vi "NF90 command interface.vi"(0 "port number in":refnum<visa-resource-name>, 1 "scaling (steps/cm)":sgl=2000.0 min=-1048575 max=1048575 step=1 format="%.2f", 2 "time out (ms)":u32=30000, 5 "commands":T2, 7 "axis":T1, 9 "enable?":bool, 11 "Error In":errorcluster, 12 "Distance":sgl format="%.2f", 13 "Speed":sgl=1.0 format="%.2f", 14 "Acceleration":u8=1 min=1 max=50 step=1) -> (4 "port number out":refnum<visa-resource-name>, 6 "Response":string, 8 "Position":sgl format="%.2f", 10 "timed out":bool, 15 "Error Out":errorcluster)   [LabVIEW 2015]
uses:
  NF90 commands.ctl
  Axis.ctl
panel:
  out "Command String":string
  in  "code":string[](array[string])=["I", "S", "A", "B", "Q", "R", "N", "V", "C", "F", "G", "H"]
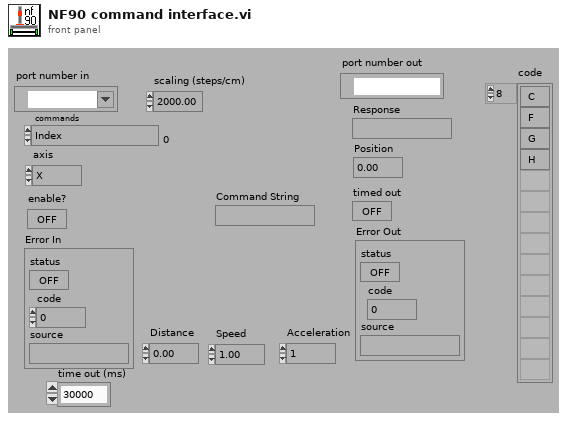
[diagram p1: front panel]
types:
  T1 = typedef "Axis.ctl" = enum16{"X", "Y", "Z"}
  T2 = typedef "NF90 commands.ctl" = enum16{"Index", "Speed", "Acceleration", "Backlash", "Quit", "Run", "Null indexes", "Verify status", "Clear program", "Computer Control", "Go", "Put Controller on Hold", "Position"}
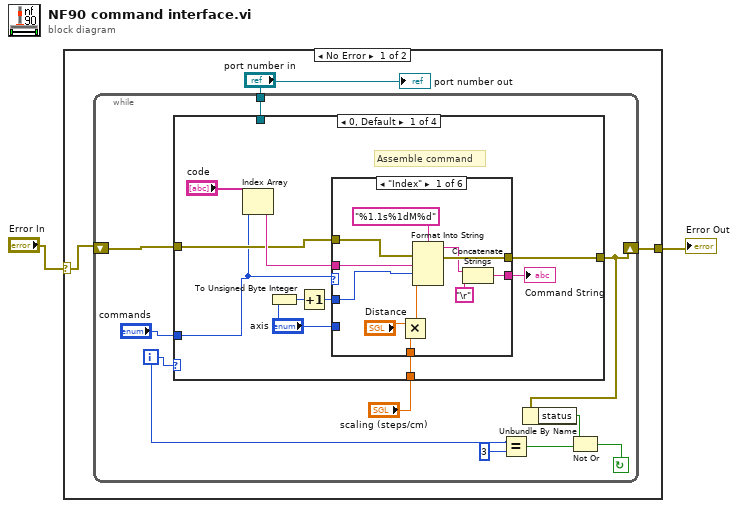
[diagram p0: block diagram]
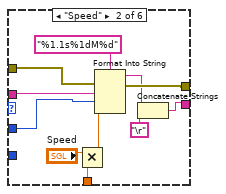
[diagram p2: hidden frame]
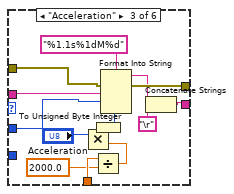
[diagram p3: hidden frame]
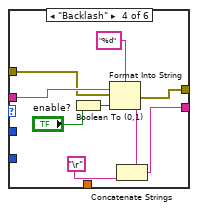
[diagram p4: hidden frame]
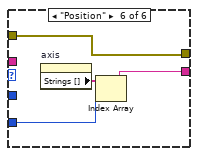
[diagram p6: hidden frame]
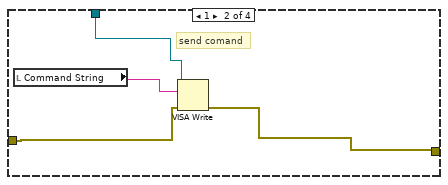
[diagram p7: hidden frame]
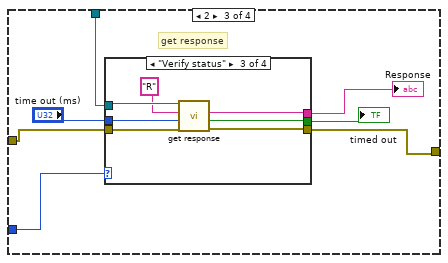
[diagram p8: hidden frame]
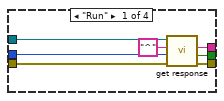
[diagram p9: hidden frame]
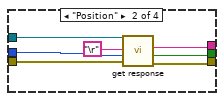
[diagram p10: hidden frame]
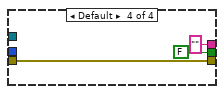
[diagram p11: hidden frame]
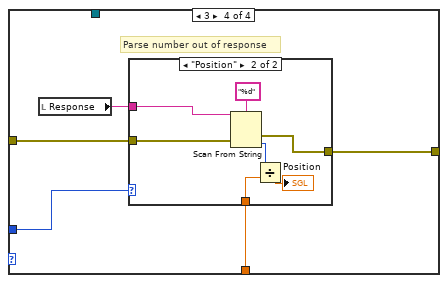
[diagram p12: hidden frame]
diagram:
  n1 = case shown="No Error" "Error In" {
    selector: "Error In" -> [w3 w125]
    tunnel: [w4 w125] -> w2
    frame No Error {
      n2 = while {
        tunnel: "port number in" -> [w13]
        shift-left: w3 -> [w14]
        shift-right: [w12] -> w4
        i -> [w15]
        stop <- w7 continue-if-true
        n3 = case shown="0, Default" w15 {
          tunnel: w14 -> [w20 w78 w86 w116]
          tunnel: [w19 w77 w84 w115] -> w12
          tunnel: w13 -> [_ w80 w87 _]
          tunnel: "commands" -> [w17 _ w83 w114]
          tunnel: "scaling (steps/cm)" -> [w16 _ _ w112]
          frame 0, Default {
            # "Assemble command"
            n4 = Index Array(array="code", index=w17) -> (element=w24:string)
            n5 = To Unsigned Byte Integer(number="axis") -> (unsigned 8bit integer=w18:u8)
            n6 = Increment(x=w18) -> (x+1=w21:u8)
            n7 = case shown="\"Index\"" w17 {
              tunnel: w24 -> [w35 w44 w58 w64 w72 _]
              tunnel: [w29 w39 w54 w69 w72 w73] -> w23
              tunnel: w21 -> [w34 w43 w57 _ _ _]
              tunnel: w20 -> [w33 w45 w59 w63 w71 w76]
              tunnel: [w32 w42 w60 w62 w71 w76] -> w19
              tunnel: "axis" -> [_ _ _ _ _ w74]
              tunnel: w16 -> [w26 w37 w51 _ _ _]
              frame "Index" {
                n8 = Multiply(x="Distance", y=w26) -> (x*y=w28:sgl)
                n9 = Format Into String(format string="%1.1s%1dM%d" ("Format String"), error in=w33, w35, w34, w28) -> (resulting string=w30:string, error out=w32:errorcluster)  [unwired: 1 in]
                n10 = Concatenate Strings(w30, "\r") -> (w29:string)
              }
              frame "Speed" {
                n11 = Multiply(x="Speed", y=w37) -> (x*y=w38:sgl)
                n12 = Format Into String(format string="%1.1s%1dM%d" ("Format String"), error in=w45, w44, w43, w38) -> (resulting string=w40:string, error out=w42:errorcluster)  [unwired: 1 in]
                n13 = Concatenate Strings(w40, "\r") -> (w39:string)
              }
              frame "Acceleration" {
                n14 = Divide(x=w51, y=sgl 2000.0) -> (x/y=w49:sgl)
                n15 = Multiply(x="Acceleration", y=w49) -> (x*y=w53:sgl)
                n16 = To Unsigned Byte Integer(number=w53) -> (unsigned 8bit integer=w48:u8)
                n17 = Format Into String(format string="%1.1s%1dM%d" ("Format String"), error in=w59, w58, w57, w48) -> (resulting string=w55:string, error out=w60:errorcluster)  [unwired: 1 in]
                n18 = Concatenate Strings(w55, "\r") -> (w54:string)
              }
              frame "Backlash" {
                n19 = Boolean To (0,1)(Boolean="enable?") -> (0, 1=w68:i16)
                n20 = Format Into String(format string="%d" ("Format String"), initial string=w64, error in=w63, w68) -> (resulting string=w65:string, error out=w62:errorcluster)
                n21 = Concatenate Strings(w65, "\r") -> (w69:string)
              }
              frame "Quit".."Put Controller on Hold", Default {
              }
              frame "Position" {
                n22 = property on="axis" class="Enum (strict)"() -> ("Strings []"=w75:string[])  [unwired: 2 in, 2 out]
                n23 = Index Array(array=w75, index=w74) -> (element=w73:string)
              }
            }
            "Command String" <- w23
          }
          frame 1 {
            # "send comand"
            n24 = local read "Command String"() -> (w79:string)
            n25 = VISA Write(VISA resource name=w80, write buffer=w79, error in (no error)=w78) -> (error out=w77:errorcluster)  [unwired: 2 out]
          }
          frame 2 {
            # "get response"
            n26 = case shown="\"Verify status\"" w83 {
              tunnel: w87 -> [w94 w101 w108 _]
              tunnel: w86 -> [w93 w100 w104 w111]
              tunnel: [w92 w98 w107 "" ("response")] -> w85
              tunnel: [w91 w99 w106 w111] -> w84
              tunnel: "time out (ms)" -> [w89 w96 w105 _]
              tunnel: [w88 w95 w103 FALSE ("timed out")] -> w81
              frame "Run" {
                n27 = call "get response.vi"("error in (no error)"=w93, "time out (ms)"=w89, "end char"="^", "port number"=w94) -> ("error out"=w91:errorcluster, "timed out"=w88:bool, "response"=w92:string)  [unwired: 4 in, 1 out]
              }
              frame "Position" {
                n28 = call "get response.vi"("error in (no error)"=w100, "time out (ms)"=w96, "end char"="\r", "port number"=w101) -> ("error out"=w99:errorcluster, "timed out"=w95:bool, "response"=w98:string)  [unwired: 4 in, 1 out]
              }
              frame "Verify status" {
                n29 = call "get response.vi"("error in (no error)"=w104, "time out (ms)"=w105, "end char"="R", "port number"=w108) -> ("error out"=w106:errorcluster, "timed out"=w103:bool, "response"=w107:string)  [unwired: 4 in, 1 out]
              }
              frame Default {
              }
            }
            "timed out" <- w81
            "Response" <- w85
          }
          frame 3 {
            # "Parse number out of response"
            n30 = local read "Response"() -> (w113:string)
            n31 = case shown="\"Position\"" w114 {
              tunnel: w116 -> [w117 w123]
              tunnel: [w117 w122] -> w115
              tunnel: w113 -> [_ w121]
              tunnel: w112 -> [_ w118]
              frame Default {
              }
              frame "Position" {
                n32 = Scan From String(format string="%d" ("Format String"), input string=w121, error in=w123) -> (error out=w122:errorcluster, output 1=w120:i32)  [unwired: 2 in, 2 out]
                n33 = Divide(x=w120, y=w118) -> (x/y=→"Position":sgl)
              }
            }
          }
        }
        n34 = Equal?(x=w15, y=3) -> (x = y?=w8:bool)
        n35 = Unbundle By Name(w12) -> ("status"=w9:bool)
        n36 = Not Or(1:w8, 2:w9) -> (0:w7:bool)
      }
      "port number out" <- "port number in"
    }
    frame Error {
    }
  }
  "Error Out" <- w2
